vi "Single Phase - 20 symmetric taps.vi"(0 "input data":fxp<+/-,18,1>[](array[numeric])=[-0.00127410888671875, 0.0, 0.0, 0.0, 0.0, 0.0, 0.0, 0.0, 0.0, 0.0, 0.0, 0.0, 0.0, 0.0, 0.0, 0.0, 0.0, 0.0, 0.0, 0.0, 0.0, 0.0, 0.0, 0.0, 0.0, 0.0, 0.0, 0.0, 0.0, 0.0, 0.0, 0.0, 0.0, 0.0, 0.0, 0.0, 0.0, 0.0, 0.0, 0.0], 7 "coefficients":fxp<+/-,18,1>[](array[numeric])=[-0.00127410888671875, 0.00325775146484375, -0.0070953369140625, 0.01354217529296875, -0.02376556396484375, 0.03955841064453125, -0.0644073486328125, 0.10701751708984375, -0.1994476318359375, 0.6322708129882812], 13 "phase":i16) -> (4 "output data":fxp<+/-,18,1>)   [LabVIEW 2019]
uses:
  <vilib>/rvi/FXPMathLib/basic elements/DSP48E/simVIs/niFpgaDsp48eSimulationState.ctl
  <vilib>/rvi/FXPMathLib/basic elements/DSP48E/subVIs/niFpgaDsp48eType.ctl
  <vilib>/rvi/FXPMathLib/basic elements/DSP48E/subVIs/niFpgaDsp48eAlumodeOpmodeCarryinselState.ctl
  <vilib>/rvi/FXPMathLib/basic elements/DSP48E/subVIs/niFpgaDsp48eUseMultiplierState.ctl
  <vilib>/rvi/FXPMathLib/basic elements/DSP48E/subVIs/niFpgaDsp48eLogicUnitModeState.ctl
  <vilib>/rvi/FXPMathLib/basic elements/DSP48E/subVIs/niFpgaDsp48eSelectPatternState.ctl
  <vilib>/rvi/FXPMathLib/basic elements/DSP48E/subVIs/niFpgaDsp48eSelectMaskState.ctl
  <vilib>/rvi/FXPMathLib/basic elements/DSP48E/subVIs/niFpgaDsp48eAutoresetState.ctl
  <vilib>/rvi/FXPMathLib/basic elements/DSP48E/simVIs/niFpgaDsp48eResets.ctl
  <vilib>/rvi/FXPMathLib/basic elements/DSP48E/simVIs/niFpgaDsp48eEnables.ctl
  <vilib>/rvi/FXPMathLib/basic elements/DSP48E/simVIs/niFpgaDsp48eRegisters.ctl
  <vilib>/rvi/FXPMathLib/basic elements/DSP48E/simVIs/niFpgaDsp48eCheckMode.vi
  <vilib>/rvi/FXPMathLib/basic elements/DSP48E/simVIs/niFpgaDsp48eReportInvalidMode.vi
  <vilib>/rvi/FXPMathLib/basic elements/DSP48E/simVIs/niFpgaDsp48eSimMultiplier.vi
  <vilib>/rvi/FXPMathLib/basic elements/DSP48E/simVIs/niFpgaDsp48eSimArithmetic.vi
  <vilib>/rvi/FXPMathLib/basic elements/DSP48E/simVIs/niFpgaDsp48eSimPatternDetect.vi
  <vilib>/rvi/FXPMathLib/basic elements/DSP48E/simVIs/niFpgaDsp48eSimP.vi
  <vilib>/rvi/FXPMathLib/basic elements/DSP48E/simVIs/niFpgaDsp48eSimUpdateState.vi
  <vilib>/rvi/FXPMathLib/basic elements/FxpDiscreteDelay/XNode/nifxpmath_DiscreteDelay.xnode
  <vilib>/rvi/FXPMathLib/basic elements/DSP48E/XNode/niFpgaDsp48e.xnode
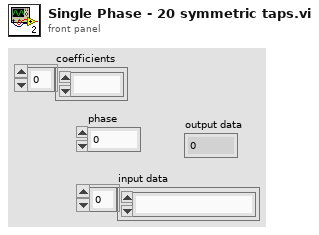
[diagram p1: front panel]
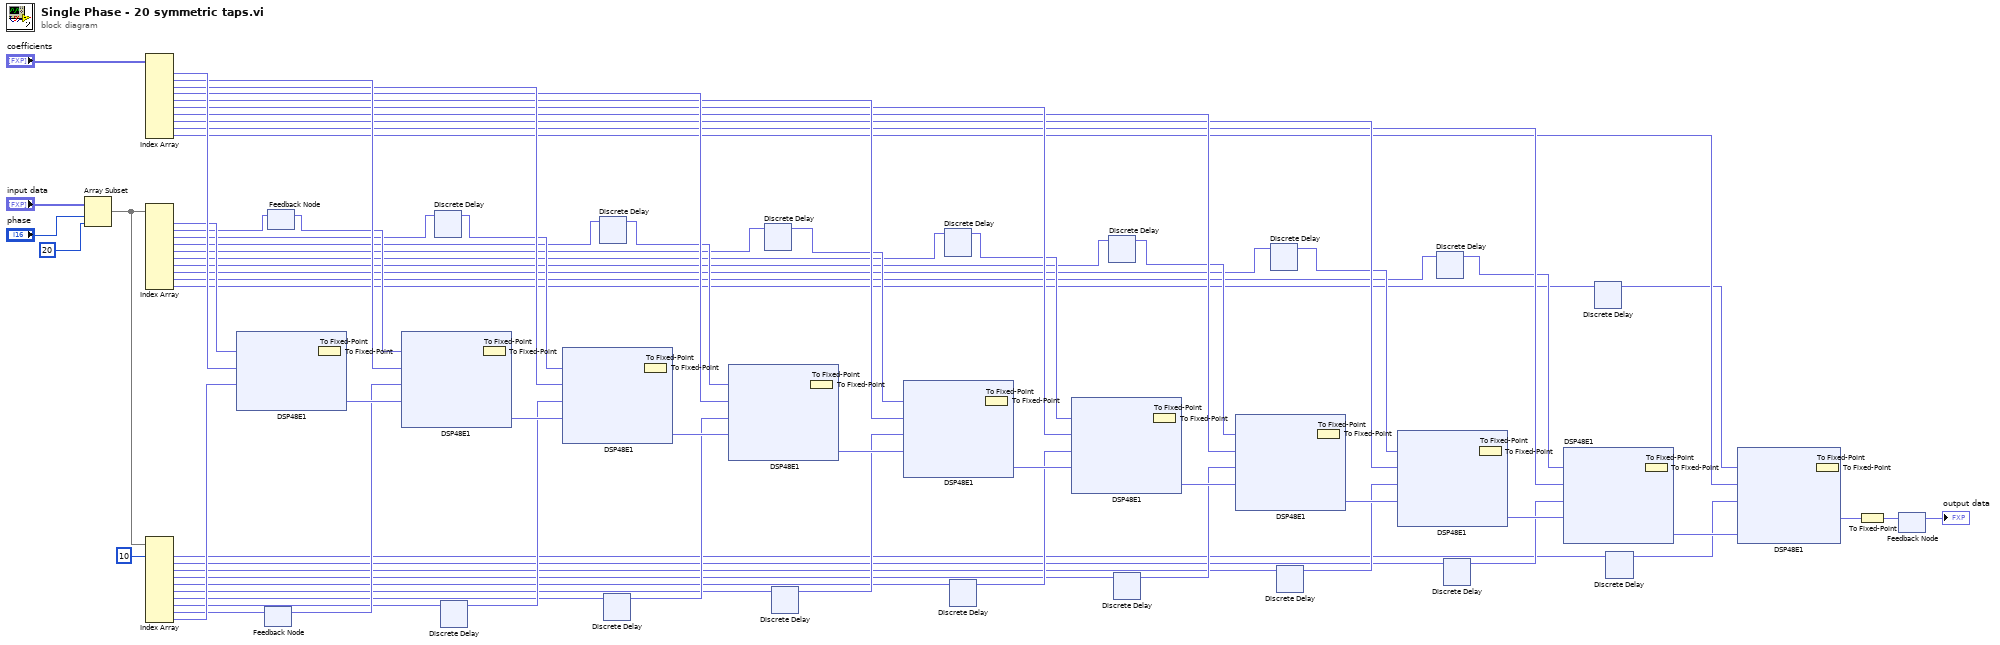
[diagram p0: block diagram]
diagram:
  n1 = Array Subset(array="input data", index="phase", length=20) -> (w73:fxp<+/-,18,1>[])
  n2 = Index Array(array="coefficients") -> (element #1=w86:fxp<+/-,18,1>, element #2=w80:fxp<+/-,18,1>, element #3=w76:fxp<+/-,18,1>, element #4=w75:fxp<+/-,18,1>, element #5=w74:fxp<+/-,18,1>, element #6=w59:fxp<+/-,18,1>, element #7=w58:fxp<+/-,18,1>, element #8=w57:fxp<+/-,18,1>, element #9=w56:fxp<+/-,18,1>, element #10=w55:fxp<+/-,18,1>)  [unwired: 10 in]
  n3 = Index Array(array=w73) -> (element #1=w85:fxp<+/-,18,1>, element #2=w70:fxp<+/-,18,1>, element #3=w53:fxp<+/-,18,1>, element #4=w51:fxp<+/-,18,1>, element #5=w49:fxp<+/-,18,1>, element #6=w47:fxp<+/-,18,1>, element #7=w45:fxp<+/-,18,1>, element #8=w43:fxp<+/-,18,1>, element #9=w41:fxp<+/-,18,1>, element #10=w39:fxp<+/-,18,1>)  [unwired: 10 in]
  n4 = Index Array(array=w73, index #1=10 ("index")) -> (element #1=w23:fxp<+/-,18,1>, element #2=w25:fxp<+/-,18,1>, element #3=w27:fxp<+/-,18,1>, element #4=w29:fxp<+/-,18,1>, element #5=w31:fxp<+/-,18,1>, element #6=w33:fxp<+/-,18,1>, element #7=w35:fxp<+/-,18,1>, element #8=w37:fxp<+/-,18,1>, element #9=w72:fxp<+/-,18,1>, element #10=w81:fxp<+/-,18,1>)  [unwired: 9 in]
  n5 = feedback-in #1(w72) -> ()
  n6 = feedback #1() -> (w71:fxp<+/-,18,1>)  [unwired: 1 in]
  n7 = feedback #2() -> (w69:fxp<+/-,18,1>)  [unwired: 1 in]
  n8 = feedback-in #2(w70) -> ()
  n9 = To Fixed-Point(number=w85) -> (fixed-point=w1:fxp<+/-,30,13>)  [unwired: 1 in]
  n10 = To Fixed-Point(number=w1) -> (fixed-point=w2:fxp<+/-,25,8>)  [unwired: 1 in]
  n11 = xnode ("DSP48E1")("a"=w2, "b"=w86, "d"=w81) -> ("pcout"=w83:fxp<+/-,48,14>)
  n12 = xnode ("Discrete Delay")("D"=w53) -> ("Q"=w52:fxp<+/-,18,1>)
  n13 = xnode ("Discrete Delay")("D"=w37) -> ("Q"=w36:fxp<+/-,18,1>)
  n14 = To Fixed-Point(number=w69) -> (fixed-point=w3:fxp<+/-,30,13>)  [unwired: 1 in]
  n15 = To Fixed-Point(number=w3) -> (fixed-point=w4:fxp<+/-,25,8>)  [unwired: 1 in]
  n16 = xnode ("DSP48E1")("a"=w4, "b"=w80, "d"=w71, "pcin"=w83) -> ("pcout"=w79:fxp<+/-,48,14>)
  n17 = xnode ("Discrete Delay")("D"=w51) -> ("Q"=w50:fxp<+/-,18,1>)
  n18 = xnode ("Discrete Delay")("D"=w35) -> ("Q"=w34:fxp<+/-,18,1>)
  n19 = To Fixed-Point(number=w52) -> (fixed-point=w5:fxp<+/-,30,13>)  [unwired: 1 in]
  n20 = To Fixed-Point(number=w5) -> (fixed-point=w6:fxp<+/-,25,8>)  [unwired: 1 in]
  n21 = xnode ("DSP48E1")("a"=w6, "b"=w76, "d"=w36, "pcin"=w79) -> ("pcout"=w78:fxp<+/-,48,14>)
  n22 = xnode ("Discrete Delay")("D"=w49) -> ("Q"=w48:fxp<+/-,18,1>)
  n23 = xnode ("Discrete Delay")("D"=w33) -> ("Q"=w32:fxp<+/-,18,1>)
  n24 = To Fixed-Point(number=w50) -> (fixed-point=w7:fxp<+/-,30,13>)  [unwired: 1 in]
  n25 = To Fixed-Point(number=w7) -> (fixed-point=w8:fxp<+/-,25,8>)  [unwired: 1 in]
  n26 = xnode ("DSP48E1")("a"=w8, "b"=w75, "d"=w34, "pcin"=w78) -> ("pcout"=w77:fxp<+/-,48,14>)
  n27 = xnode ("Discrete Delay")("D"=w47) -> ("Q"=w46:fxp<+/-,18,1>)
  n28 = xnode ("Discrete Delay")("D"=w31) -> ("Q"=w30:fxp<+/-,18,1>)
  n29 = To Fixed-Point(number=w48) -> (fixed-point=w9:fxp<+/-,30,13>)  [unwired: 1 in]
  n30 = To Fixed-Point(number=w9) -> (fixed-point=w10:fxp<+/-,25,8>)  [unwired: 1 in]
  n31 = xnode ("DSP48E1")("a"=w10, "b"=w74, "d"=w32, "pcin"=w77) -> ("pcout"=w60:fxp<+/-,48,14>)
  n32 = xnode ("Discrete Delay")("D"=w45) -> ("Q"=w44:fxp<+/-,18,1>)
  n33 = xnode ("Discrete Delay")("D"=w29) -> ("Q"=w28:fxp<+/-,18,1>)
  n34 = To Fixed-Point(number=w46) -> (fixed-point=w11:fxp<+/-,30,13>)  [unwired: 1 in]
  n35 = To Fixed-Point(number=w11) -> (fixed-point=w12:fxp<+/-,25,8>)  [unwired: 1 in]
  n36 = xnode ("DSP48E1")("a"=w12, "b"=w59, "d"=w30, "pcin"=w60) -> ("pcout"=w61:fxp<+/-,48,14>)
  n37 = xnode ("Discrete Delay")("D"=w43) -> ("Q"=w42:fxp<+/-,18,1>)
  n38 = xnode ("Discrete Delay")("D"=w27) -> ("Q"=w26:fxp<+/-,18,1>)
  n39 = To Fixed-Point(number=w44) -> (fixed-point=w13:fxp<+/-,30,13>)  [unwired: 1 in]
  n40 = To Fixed-Point(number=w13) -> (fixed-point=w14:fxp<+/-,25,8>)  [unwired: 1 in]
  n41 = xnode ("DSP48E1")("a"=w14, "b"=w58, "d"=w28, "pcin"=w61) -> ("pcout"=w62:fxp<+/-,48,14>)
  n42 = xnode ("Discrete Delay")("D"=w41) -> ("Q"=w40:fxp<+/-,18,1>)
  n43 = xnode ("Discrete Delay")("D"=w25) -> ("Q"=w24:fxp<+/-,18,1>)
  n44 = To Fixed-Point(number=w42) -> (fixed-point=w15:fxp<+/-,30,13>)  [unwired: 1 in]
  n45 = To Fixed-Point(number=w15) -> (fixed-point=w16:fxp<+/-,25,8>)  [unwired: 1 in]
  n46 = xnode ("DSP48E1")("a"=w16, "b"=w57, "d"=w26, "pcin"=w62) -> ("pcout"=w63:fxp<+/-,48,14>)
  n47 = xnode ("Discrete Delay")("D"=w39) -> ("Q"=w38:fxp<+/-,18,1>)
  n48 = xnode ("Discrete Delay")("D"=w23) -> ("Q"=w22:fxp<+/-,18,1>)
  n49 = To Fixed-Point(number=w40) -> (fixed-point=w17:fxp<+/-,30,13>)  [unwired: 1 in]
  n50 = To Fixed-Point(number=w17) -> (fixed-point=w18:fxp<+/-,25,8>)  [unwired: 1 in]
  n51 = xnode ("DSP48E1")("a"=w18, "b"=w56, "d"=w24, "pcin"=w63) -> ("pcout"=w64:fxp<+/-,48,14>)
  n52 = To Fixed-Point(number=w38) -> (fixed-point=w19:fxp<+/-,30,13>)  [unwired: 1 in]
  n53 = To Fixed-Point(number=w19) -> (fixed-point=w20:fxp<+/-,25,8>)  [unwired: 1 in]
  n54 = xnode ("DSP48E1")("a"=w20, "b"=w55, "d"=w22, "pcin"=w64) -> ("p"=w21:fxp<+/-,48,14>)
  n55 = To Fixed-Point(number=w21) -> (fixed-point=w68:fxp<+/-,18,1>)  [unwired: 1 in]
  n56 = feedback-in #3(w68) -> ()
  n57 = feedback #3() -> (→"output data":fxp<+/-,18,1>)  [unwired: 1 in]
